vi "test trace.vi"   [LabVIEW 2009]
uses:
  POLARIS BME DG.lvlib
types:
  T1 = enum16{"Trace", "SetPath", "NewFile?", "WriteToFile", "StartTrace", "StopTrace"}
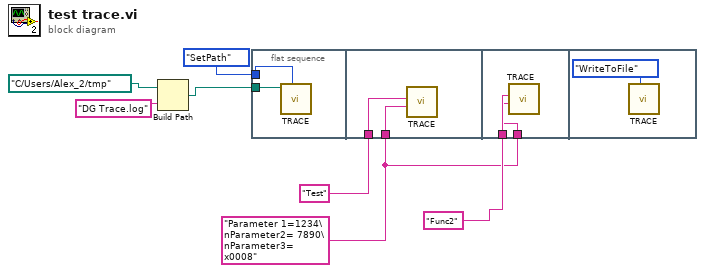
[diagram p0: block diagram]
diagram:
  w1 = "Parameter 1=1234\nParameter2= 7890\nParameter3= x0008" ("Parameter String")
  n1 = Build Path(base path=path "C:/Users/Alex_2/tmp" ("TraceFile"), name or relative path="DG Trace.log") -> (appended path=w5:path)
  n2 = flat-sequence {
    tunnel: T1."SetPath" ("Mode") -> [w9]
    tunnel: w5 -> [w8]
    tunnel: "Test" ("Function") -> [w11]
    tunnel: w1 -> [w10]
    tunnel: "Func2" ("Function") -> [w13]
    tunnel: w1 -> [w12]
    frame #0 {
      n3 = call "TRACE.vi"("Mode"=w9, "TraceFile"=w8) -> ()  [unwired: 10 in]
    }
    frame #1 {
      n4 = call "TRACE.vi"("Parameter String"=w10, "Function"=w11) -> ()  [unwired: 10 in]
    }
    frame #2 {
      n5 = call "TRACE.vi"("Parameter String"=w12, "Function"=w13) -> ()  [unwired: 10 in]
    }
    frame #3 {
      n6 = call "TRACE.vi"("Mode"=T1."WriteToFile") -> ()  [unwired: 11 in]
    }
  }
